vi "Channel Command Engine.vi"(8 "error in":errorcluster, 11 "State Variables":T1={"TCP Refs"={"Connection List"=refnum, "listener ID"=refnum}, "Stop"=refnum, "Top VI"=refnum, "Parameters"={"Properties"={"Name"="", "CAN"={"Database File"=path "", "CAN Interface"=enum."CAN0", "Baud Rate"=0, "Diagnostic Protocol"=enum."GMLAN", "Transport Protocol"=enum."ISO TP - Normal Mode", "Transmit ID"=0, "Receive ID"=0, "Transmit Extension"=0, "Receive Extension"=0, "Receive UUDT ID"=0, "Enable Stream"=TRUE, "VW TP Channel ID"=0, "Security"={"Source DLL Path"=path "", "Security Level"=1, "Target DLL Path"=path ""}, "Fill Frame"=FALSE, "Fill Byte"=255, "Termination"=FALSE}, "FPGA Settings"={"RT Bitfile Path"=path "", "RIO Device"=0, "Enable"=FALSE}, "Reads"=[], "Frames Lookup"=variant, "Writes"=[], "DPIDs"=[], "DPID Lookup"=variant, "DTC descriptor"={"DTC Byte Length"=2, "Status Byte Length"=1, "Add Data Byte Length"=1, "Byte Order"=enum."Motorola"}}, "ChanRefs"={"ToVS.Reads"={"Name"="", "Write to VS Engine FIFO"=refnum, "Pairs"={"Refs"=[], "Values"=[]}}, "ToVS.DTCs"={"Name"="", "Write to VS Engine FIFO"=refnum, "Pairs"={"Refs"=[], "Values"=[]}}, "ToVS.DTCCount"={"Name"="", "Write to VS Engine FIFO"=refnum, "Pairs"={"Refs"=[], "Values"=[]}}, "ToVS.Status"={"Name"="", "Write to VS Engine FIFO"=refnum, "Pairs"={"Refs"=[], "Values"=[]}}, "FromVS.Writes"={"Name"="", "Read from VS Engine FIFO"=refnum, "Pairs"={"Refs"=[], "Values"=[]}}, "Cmds"={"Name"="", "Write to VS Engine FIFO"=refnum, "Read from VS Engine FIFO"=refnum, "Pairs"={"Chan Refs"=[], "Prev. Values"=[]}}}}, "ADCS Connection"={"Diag CAN Handle"=0, "Transport Protocol"=enum."ISO TP - Normal Mode", "Receive Address Extension"=0, "Transmit Address Extension"=0, "Receive CAN Id"=0, "Transmit CAN Id"=0, "Diag CAN Queue"=refnum, "Log Frames ?"=FALSE, "My TP Address"=0, "Other TP Address"=0, "T1"=0, "T2"=0, "T3"=0, "T4"=0, "Tx SN"=0, "Block Size"=0, "Rx SN"=0, "VW TP Initialized?"=FALSE, "Tx block no"=0, "baud rate"=0, "Interface"="", "Channel Diag CAN Handle"=0, "UDP Connection ID"=refnum, "TCP Connection ID"=refnum, "Target IP Addr"=0, "Source Address"=0, "Target Address"=0, "Send Header NACK?"=FALSE, "DLL Handle"=0, "NAD"=0, "Time Stamp read first"=0.0, "Time Stamp read last"=0.0, "Time Stamp write first"=0.0, "Time Stamp write last"=0.0, "Time Stamp write"=0.0, "Time Stamp read"=0.0}, "XNET References"={"Database"="", "GMLAN DPID Session"="", "Cluster"=""}, "BufferedCmds"=refnum, "XNETEngine (GMLAN)"=refnum} {"Parameters"."ChanRefs"."Cmds"."Pairs"."Chan Refs" format="%.0x"; "Parameters"."ChanRefs"."ToVS.Status"."Pairs"."Refs" format="%.0x"; "Parameters"."ChanRefs"."ToVS.DTCCount"."Pairs"."Refs" format="%.0x"; "Parameters"."ChanRefs"."ToVS.DTCs"."Pairs"."Refs" format="%.0x"; "Parameters"."ChanRefs"."ToVS.Reads"."Pairs"."Refs" format="%.0x"; "Parameters"."Properties"."Writes"."Signals"."Byte Order" items=["Little Endian", "Big Endian"]; "Parameters"."Properties"."Writes"."Signals"."Data Type" items=["Signed", "Unsigned", "IEEE Float"]; "Parameters"."Properties"."CAN"."Fill Byte" format="%.0x"; "Parameters"."Properties"."CAN"."VW TP Channel ID" format="%.0x"; "Parameters"."Properties"."CAN"."Receive UUDT ID" format="%.0x"; "Parameters"."Properties"."CAN"."Receive Extension" format="%.0x"; "Parameters"."Properties"."CAN"."Transmit Extension" format="%.0x"; "Parameters"."Properties"."CAN"."Receive ID" format="%.0x"; "Parameters"."Properties"."CAN"."Transmit ID" format="%.0x"; "Parameters"."Properties"."Reads"."Signals"."Byte Order" items=["Little Endian", "Big Endian"]; "Parameters"."Properties"."Reads"."Signals"."Data Type" items=["Signed", "Unsigned", "IEEE Float"]}) -> (0 "error out":errorcluster)   [LabVIEW 2015, in "Diagnostics Addon Engine.lvlib"]
uses:
  Diagnostics Addon Engine.lvlib
  Types/State Variables.ctl
  Types/TCP Refs.ctl
  STM/STM Lookup Table Ref.ctl
  Stop FG/Stop Global Ref.ctl
  Types/Main Configuration.ctl
  Shared/Types/Section Properties.ctl
  Shared/Types/CAN Configuration.ctl
  Shared/Types/CAN Interface.ctl
  Shared/Types/Diagnostic Protocols.ctl
  Shared/Types/Transport Protocols.ctl
  Shared/Types/Security.ctl
  Shared/Types/FPGA Bitfile Settings.ctl
  Shared/Types/Common Frame Parameters.ctl
  Shared/Types/MessageType Selector.ctl
  Shared/Types/Signal Parameters.ctl
  Shared/Types/DPID Parameters.ctl
  Shared/Types/DPID Periodic Rate.ctl
  Shared/Types/DTC Descriptor Parameters.ctl
  Types/VS Data Channels.ctl
  Inline Async API/Controls/Write To VS Engine.ctl
  <vilib>/NI Veristand/Custom Device API/Data Reference.ctl
  Inline Async API/Controls/Read From VS Engine.ctl
  <vilib>/NI Veristand/Custom Device API/Block Data Reference.ctl
  Inline Async API/Controls/ReadWrite Data.ctl
  <vilib>/Automotive Diagnostic Command Set/Diagnostic Transport.llb/Diag Reference.ctl
  <vilib>/Automotive Diagnostic Command Set/Diagnostic Transport.llb/Transport Protocol Selector.ctl
  <vilib>/Automotive Diagnostic Command Set/Diagnostic Transport.llb/Diag CAN Frame Log.ctl
  Types/XNET References.ctl
  <vilib>/NI/AMC/Message Queue.ctl
  <vilib>/NI/AMC/Message.ctl
  <vilib>/NI/Tools/Keyed Array/KeyedArray.ctl
  Stop FG/Stop Global Commands.ctl
  Shared/Types/Channel Commands Enum.ctl
  Shared/Types/Memory Command Parameters.ctl
  Shared/Types/PassThru Channel Based Command Parameters.ctl
  Shared/Types/ReadDTCbyDTCNumber Parameters.ctl
  Shared/Types/Communication Parameters.ctl
  Shared/Types/Input Output Cmd Parameters.ctl
  GMLAN/_SubVIs/ReadFailureRecordData_readFailureRecordParameters_failureRecordIdentifier.ctl
  <vilib>/NI/AMC/Update Message Routing Info.vi
  <vilib>/NI/AMC/Create Multiple Messages.vi
  <vilib>/NI/AMC/Create Single Message.vi
  <vilib>/NI/AMC/Send Message.vi
  Error Handling API/Error Handling API.lvlib
  Stop FG/Stop FG.lvlib
  Shared/Diagnostics Addon Shared.lvlib
  <vilib>/NI/AMC/AMC.lvlib
  GMLAN/GMLAN.lvlib
  <vilib>/NI Veristand/Custom Device API/Custom Device API.lvlib
  <vilib>/NI/Tools/Keyed Array/Tools_KeyedArray.lvlib
  <vilib>/addons/Automotive Diagnostic Command Set/NI_Automotive Diagnostic Command Set.lvlib
  Inline Async API/Inline Async API.lvlib
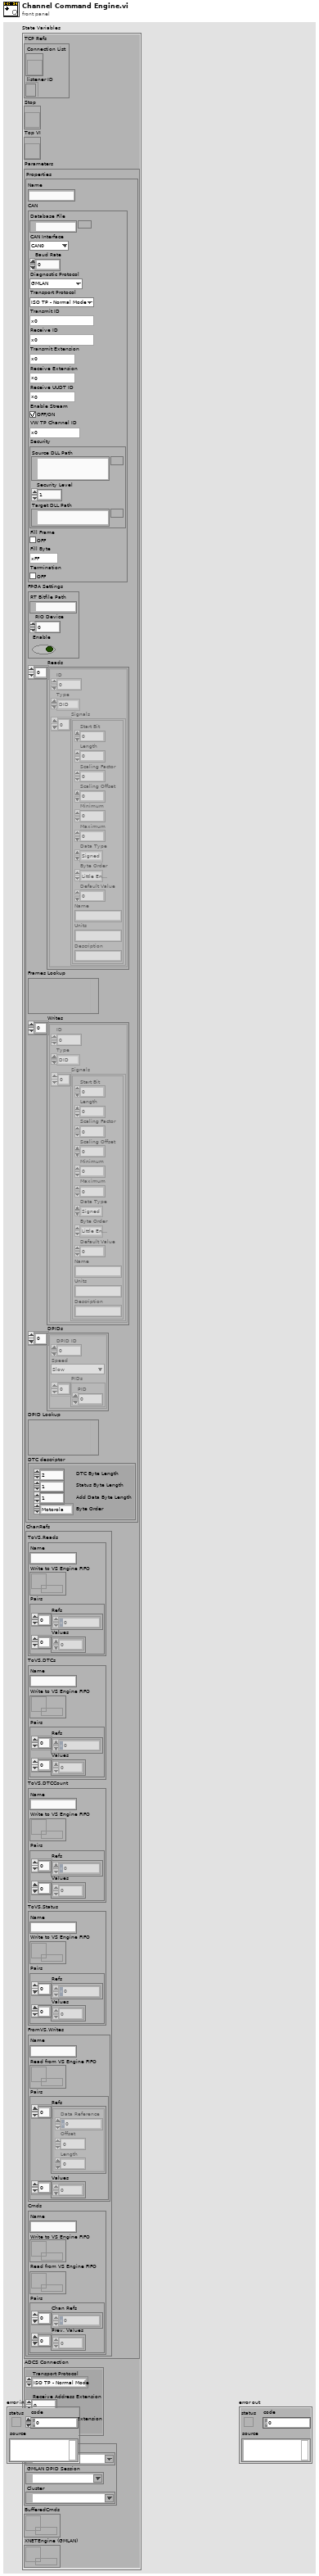
[diagram p1: front panel]
types:
  T1 = typedef "Diagnostics Addon Engine.lvlib/State Variables.ctl" = cluster{"TCP Refs":T2, "Stop":T4, "Top VI":refnum<vi>, "Parameters":T5, "ADCS Connection":T25, "XNET References":T27, "BufferedCmds":T28, "XNETEngine (GMLAN)":T28}
  T2 = typedef "Diagnostics Addon Engine.lvlib/TCP Refs.ctl" = cluster{"Connection List":T3, "listener ID":refnum<k5>}
  T3 = typedef "Diagnostics Addon Engine.lvlib/STM Lookup Table Ref.ctl" = refnum<vi>
  T4 = typedef "Diagnostics Addon Engine.lvlib/Stop FG.lvlib/Stop Global Ref.ctl" = refnum<vi>
  T5 = typedef "Diagnostics Addon Engine.lvlib/Main Configuration.ctl" = cluster{"Properties":T6, "ChanRefs":T19}
  T6 = typedef "Diagnostics Addon Shared.lvlib/Section Properties.ctl" = cluster{"Name":string, "CAN":T7, "FPGA Settings":T12, "Reads":T13[], "Frames Lookup":variant, "Writes":T13[], "DPIDs":T16[], "DPID Lookup":variant, "DTC descriptor":T18}
  T7 = typedef "Diagnostics Addon Shared.lvlib/CAN Configuration.ctl" = cluster{"Database File":path, "CAN Interface":T8, "Baud Rate":u32, "Diagnostic Protocol":T9, "Transport Protocol":T10, "Transmit ID":u32, "Receive ID":u32, "Transmit Extension":u8, "Receive Extension":u8, "Receive UUDT ID":u32, "Enable Stream":bool, "VW TP Channel ID":u32, "Security":T11, "Fill Frame":bool, "Fill Byte":u8, "Termination":bool}
  T8 = typedef "Diagnostics Addon Shared.lvlib/CAN Interface.ctl" = enum16{"CAN0", "CAN1", "CAN2", "CAN3", "CAN4", "CAN5", "CAN6", "CAN7", "CAN8", "CAN9", "CAN10", "CAN11", "CAN12", "CAN13", "CAN14", "CAN15", "CAN16", "CAN17", "CAN18", "CAN19", "CAN20", "CAN21", "CAN22", "CAN23", "CAN24", "CAN25", "CAN26", "CAN27", "CAN28", "CAN29", "CAN30", "CAN31", "CAN32", "CAN33", "CAN34", "CAN35", "CAN36", "CAN37", "CAN38", "CAN39", "CAN40", "CAN41", "CAN42", "CAN43", "CAN44", "CAN45", "CAN46", "CAN47", "CAN48", "CAN49", "CAN50", "CAN51", "CAN52", "CAN53", "CAN54", "CAN55", "CAN56", "CAN57", "CAN58", "CAN59", "CAN60", "CAN61", "CAN62", "CAN63", "CAN 256 (Virtual)", "CAN 257 (Virtual)"}
  T9 = typedef "Diagnostics Addon Shared.lvlib/Diagnostic Protocols.ctl" = enum16{"GMLAN", "KWP-2000", "UDS"}
  T10 = typedef "Diagnostics Addon Shared.lvlib/Transport Protocols.ctl" = enum16{"ISO TP - Normal Mode", "ISO TP - Mixed Mode", "VW TP 2.0", "Diagnostics on IP"}
  T11 = typedef "Diagnostics Addon Shared.lvlib/Security.ctl" = cluster{"Source DLL Path":path, "Security Level":u8, "Target DLL Path":path}
  T12 = typedef "Diagnostics Addon Shared.lvlib/FPGA Bitfile Settings.ctl" = cluster{"RT Bitfile Path":path, "RIO Device":u16, "Enable":bool}
  T13 = typedef "Diagnostics Addon Shared.lvlib/Common Frame Parameters.ctl" = cluster{"ID":u32, "Type":T14, "Signals":T15[]}
  T14 = typedef "Diagnostics Addon Shared.lvlib/MessageType Selector.ctl" = enum16{"DID", "CDID", "PID", "CPID", "Write Memory", "Read Memory", "DTC Control", "IO Cmd", "IO Resp", "Routine Start Cmd", "Routine Start Resp", "Routine Status Cmd", "Routine Status Resp", "Routine Stop Cmd", "Routine Stop Resp"}
  T15 = typedef "Diagnostics Addon Shared.lvlib/Signal Parameters.ctl" = cluster{"Start Bit":u8, "Length":u8, "Scaling Factor":dbl, "Scaling Offset":dbl, "Minimum":dbl, "Maximum":dbl, "Data Type":u32, "Byte Order":u32, "Default Value":dbl, "Name":string, "Units":string, "Description":string}
  T16 = typedef "Diagnostics Addon Shared.lvlib/DPID Parameters.ctl" = cluster{"DPID ID":u8, "Speed":T17, "PIDs":u16[]}
  T17 = typedef "Diagnostics Addon Shared.lvlib/DPID Periodic Rate.ctl" = enum16{"Slow", "Medium", "Fast"}
  T18 = typedef "Diagnostics Addon Shared.lvlib/DTC Descriptor Parameters.ctl" = cluster{"DTC Byte Length":i32, "Status Byte Length":i32, "Add Data Byte Length":i32, "Byte Order":enum16{"Motorola", "Intel"}}
  T19 = typedef "Diagnostics Addon Engine.lvlib/VS Data Channels.ctl" = cluster{"ToVS.Reads":T20, "ToVS.DTCs":T20, "ToVS.DTCCount":T20, "ToVS.Status":T20, "FromVS.Writes":T22, "Cmds":T24}
  T20 = typedef "Diagnostics Addon Engine.lvlib/Inline Async API.lvlib/Write To VS Engine.ctl" = cluster{"Name":string, "Write to VS Engine FIFO":refnum<k33>, "Pairs":cluster{"Refs":T21[], "Values":dbl[]}}
  T21 = typedef "Custom Device API.lvlib/Data Reference.ctl" = i32
  T22 = typedef "Diagnostics Addon Engine.lvlib/Inline Async API.lvlib/Read From VS Engine.ctl" = cluster{"Name":string, "Read from VS Engine FIFO":refnum<k33>, "Pairs":cluster{"Refs":T23[], "Values":dbl[]}}
  T23 = typedef "Custom Device API.lvlib/Block Data Reference.ctl" = cluster{"Data Reference":T21, "Offset":u64, "Length":u64}
  T24 = typedef "Diagnostics Addon Engine.lvlib/Inline Async API.lvlib/ReadWrite Data.ctl" = cluster{"Name":string, "Write to VS Engine FIFO":refnum<k33>, "Read from VS Engine FIFO":refnum<k33>, "Pairs":cluster{"Chan Refs":T21[], "Prev. Values":dbl[]}}
  T25 = typedef "NI_Automotive Diagnostic Command Set.lvlib/Diag Reference.ctl" = cluster{"Diag CAN Handle":u32, "Transport Protocol":T26, "Receive Address Extension":u8, "Transmit Address Extension":u8, "Receive CAN Id":u32, "Transmit CAN Id":u32, "Diag CAN Queue":refnum<queue>, "Log Frames ?":bool, "My TP Address":u8, "Other TP Address":u8, "T1":u16, "T2":u16, "T3":u16, "T4":u16, "Tx SN":u8, "Block Size":u8, "Rx SN":u8, "VW TP Initialized?":bool, "Tx block no":u8, "baud rate":u32, "Interface":string, "Channel Diag CAN Handle":u32, "UDP Connection ID":refnum<k16>, "TCP Connection ID":refnum<k5>, "Target IP Addr":u32, "Source Address":u16, "Target Address":u16, "Send Header NACK?":bool, "DLL Handle":u32, "NAD":u8, "Time Stamp read first":dbl, "Time Stamp read last":dbl, "Time Stamp write first":dbl, "Time Stamp write last":dbl, "Time Stamp write":dbl, "Time Stamp read":dbl}
  T26 = typedef "NI_Automotive Diagnostic Command Set.lvlib/Transport Protocol Selector.ctl" = enum16{"ISO TP - Normal Mode", "ISO TP - Mixed Mode", "VW TP 2.0", "Diagnostics on IP", "ISO TP LIN"}
  T27 = typedef "Diagnostics Addon Engine.lvlib/XNET References.ctl" = cluster{"Database":refnum<k21>, "GMLAN DPID Session":refnum<k21>, "Cluster":refnum<k21>}
  T28 = typedef "AMC.lvlib/Message Queue.ctl" = refnum<queue>
  T29 = typedef "Diagnostics Addon Engine.lvlib/Stop FG.lvlib/Stop Global Commands.ctl" = enum16{"Write", "Read", "Reset"}
  T30 = typedef "Diagnostics Addon Shared.lvlib/Channel Commands Enum.ctl" = enum8{"None", "EnableDiagnosticSession", "DisableDiagnosticSession", "ReadDataIdentifiers", "ReadDataIdentifier", "WriteDataIndentifier", "ReadPIDsOnDemand", "ReadPIDOnDemand", "WriteCPID", "WriteMemory", "ReadMemory", "ReadDTCs", "ClearDTCs", "ControlDTC", "ForceTesterPresent", "DisableNormalCommunication", "ReturnToNormalMode", "InputOutputControl", "StartRoutine", "RequestRoutineStatus", "StopRoutine", "ECUReset", "UnlockECU", "ClearSuccessBit", "ConfigureandStartPIDs", "StopPIDs", "StartDTCs", "EnableChangeDTCCount", "DisableChangeDTCCount", "ReadFailureRecordParameters", "PassThru Channel Based"}
  T31 = typedef "Diagnostics Addon Shared.lvlib/Memory Command Parameters.ctl" = cluster{"Address":u64, "Service Type":u32, "Address Length":u8, "Size Length":u8}
  T32 = typedef "Diagnostics Addon Shared.lvlib/PassThru Channel Based Command Parameters.ctl" = cluster{"Service":u64, "Service Length":u8, "Data Length":u32, "Response Required":bool}
  T33 = typedef "Diagnostics Addon Shared.lvlib/ReadDTCbyDTCNumber Parameters.ctl" = cluster{"DTC":u16, "FailTypeByte":u8}
  T34 = typedef "Diagnostics Addon Shared.lvlib/Communication Parameters.ctl" = cluster{"Type":u8, "CommType":u8}
  T35 = typedef "Diagnostics Addon Shared.lvlib/Input Output Cmd Parameters.ctl" = cluster{"ID":u16, "Mode":u8}
  T36 = typedef "GMLAN.lvlib/ReadFailureRecordData_readFailureRecordParameters_failureRecordIdentifier.ctl" = cluster{"failureRecordNumber":u8, "DTC ID":u16, "DTCFailureType":u8}
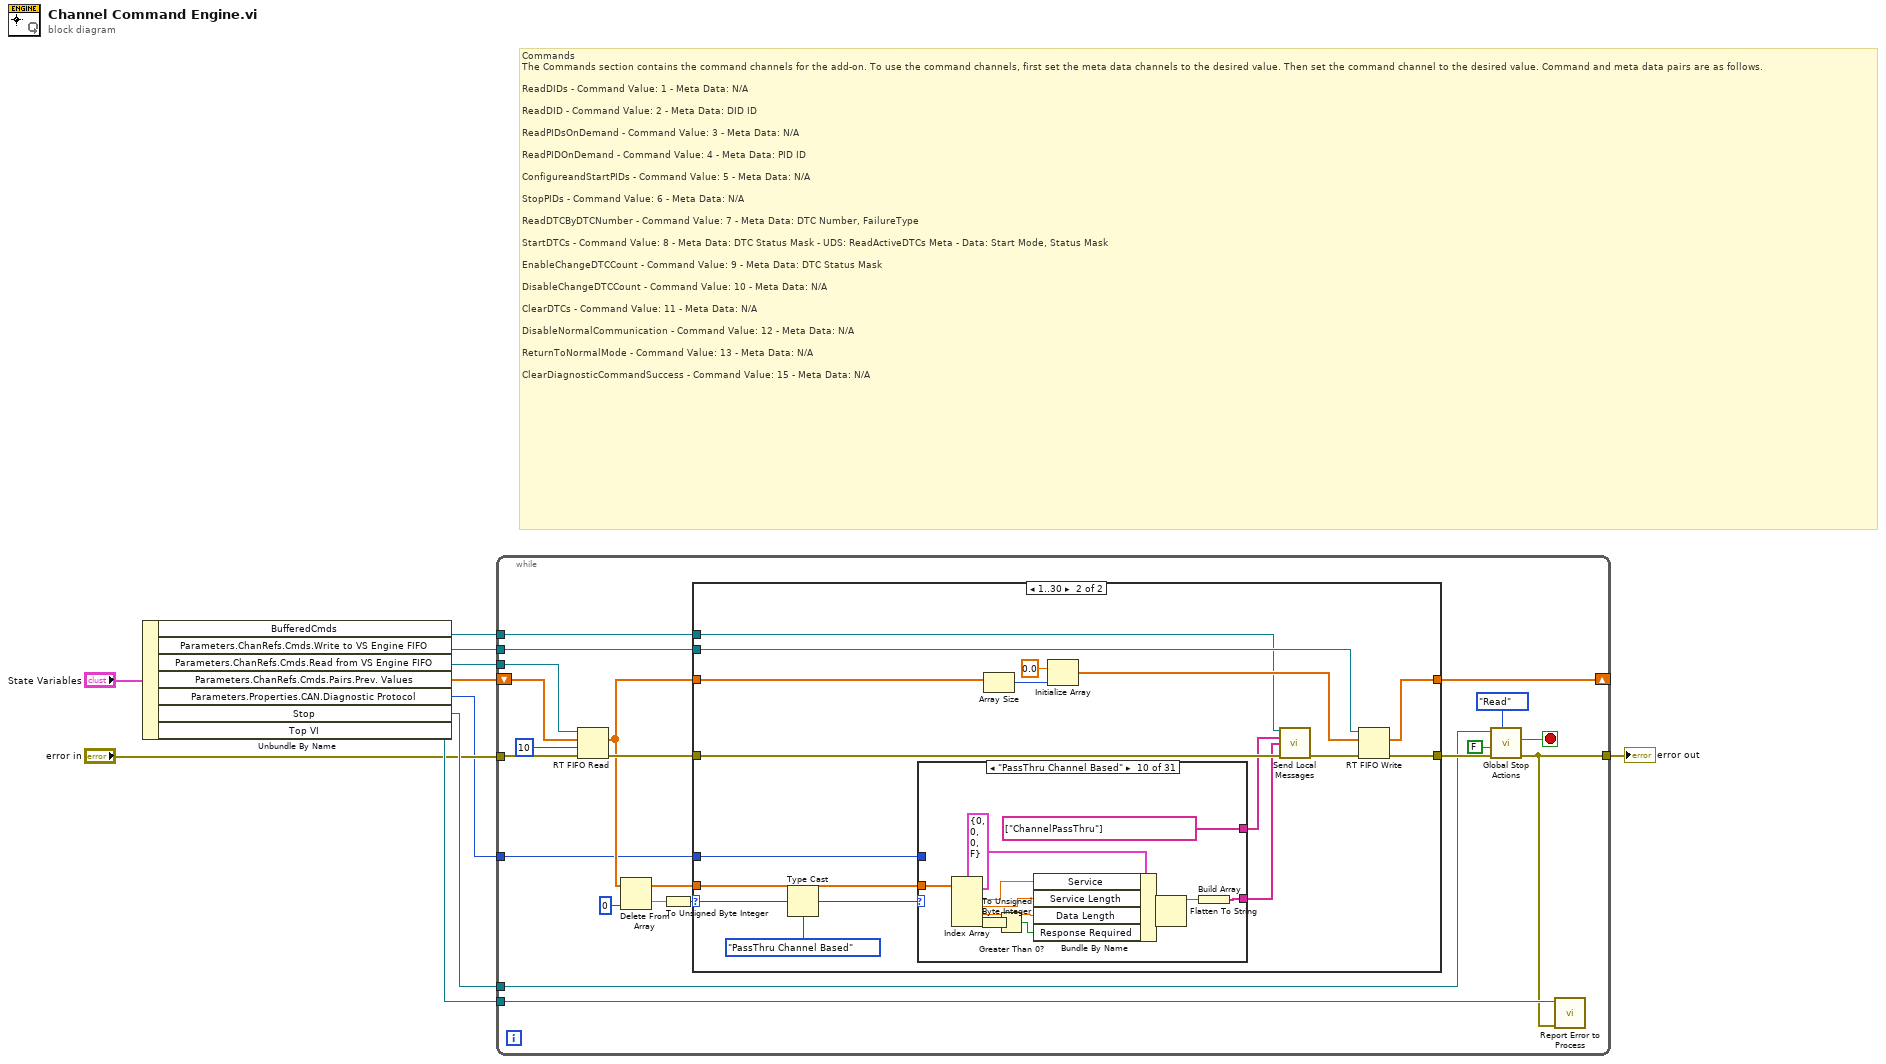
[diagram p0: block diagram]
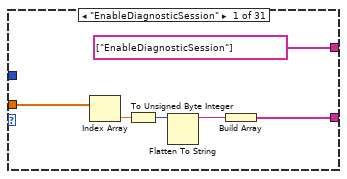
[diagram p3: hidden frame]
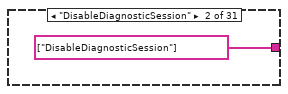
[diagram p4: hidden frame]
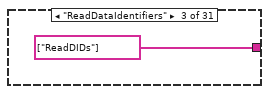
[diagram p5: hidden frame]
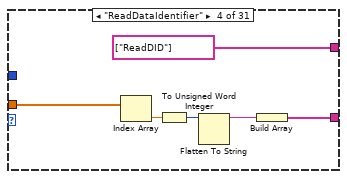
[diagram p6: hidden frame]
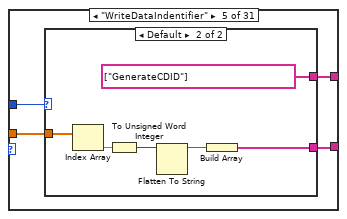
[diagram p7: hidden frame]
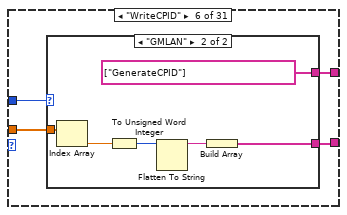
[diagram p9: hidden frame]
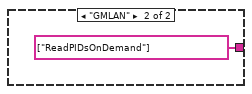
[diagram p12: hidden frame]
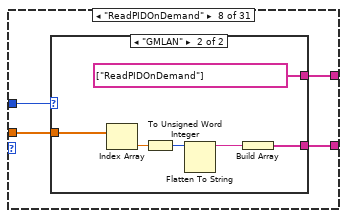
[diagram p13: hidden frame]
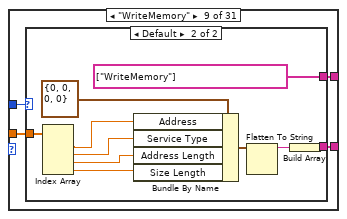
[diagram p15: hidden frame]
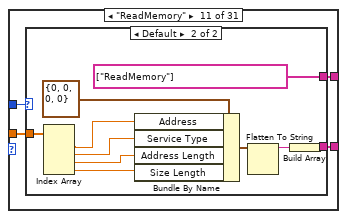
[diagram p17: hidden frame]
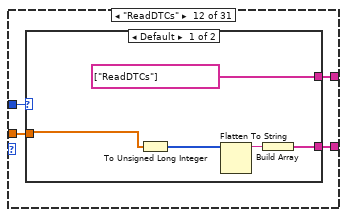
[diagram p19: hidden frame]
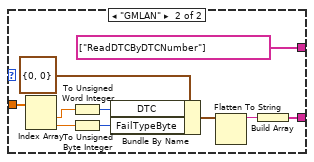
[diagram p20: hidden frame]
diagram:
  # "Commands\nThe Commands section contains the command channels for the add-on. To use the command channels, first set the meta data channels to the desired value. Then set the command channel to the desired value. Command and meta data pairs are as follows.\n\nReadDIDs - Command Value: 1 - Meta Data: N/A\n\nReadDID - Command Value: 2 - Meta Data: DID ID\n\nReadPIDsOnDemand - Command Value: 3 - Meta Data: N/A\n\nReadPIDOnDemand - Command Value: 4 - Meta Data: PID ID\n\nConfigureandStartPIDs - Command Value: 5 - Meta Data: N/A\n\nStopPIDs - Command Value: 6 - Meta Data: N/A\n\nReadDTCByDTCNumber - Command Value: 7 - Meta Data: DTC Number, FailureType\n\nStartDTCs - Command Value: 8 - Meta Data: DTC Status Mask - UDS: ReadActiveDTCs Meta - Data: Start Mode, Status Mask\n\nEnableChangeDTCCount - Command Value: 9 - Meta Data: DTC Status Mask\n\nDisableChangeDTCCount - Command Value: 10 - Meta Data: N/A\n\nClearDTCs - Command Value: 11 - Meta Data: N/A\n\nDisableNormalCommunication - Command Value: 12 - Meta Data: N/A\n\nReturnToNormalMode - Command Value: 13 - Meta Data: N/A\n\nClearDiagnosticCommandSuccess - Command Value: 15 - Meta Data: N/A"
  n1 = Unbundle By Name("State Variables") -> ("BufferedCmds"=w2:T28, "Parameters.ChanRefs.Cmds.Write to VS Engine FIFO"=w3:refnum<k33>, "Parameters.ChanRefs.Cmds.Read from VS Engine FIFO"=w5:refnum<k33>, "Parameters.ChanRefs.Cmds.Pairs.Prev. Values"=w4:dbl[], "Parameters.Properties.CAN.Diagnostic Protocol"=w1:T9, "Stop"=w9:T4, "Top VI"=w8:refnum<vi>)
  n2 = while {
    tunnel: w5 -> [w25]
    shift-right: [w23] -> _
    shift-left: w4 -> [w24]
    tunnel: w9 -> [w18]
    tunnel: w8 -> [w17]
    tunnel: [w16] -> w7
    tunnel: "error in" -> [w14]
    tunnel: w3 -> [w13]
    tunnel: w2 -> [w12]
    tunnel: w1 -> [w11]
    stop <- w15 stop-if-true
    n3 = RT FIFO Read(0:w25, 1:w24, 2:10 ("timeout in ms (0)"), 3:w14) -> (9:w26:dbl[], 11:w31:errorcluster)  [unwired: 3 out]
    n4 = Delete From Array(array=w26, index=0) -> (deleted portion=w29:dbl, array with subset deleted=w27:dbl[])  [unwired: 1 in]
    n5 = To Unsigned Byte Integer(number=w29) -> (unsigned 8bit integer=w28:u8)
    n6 = case shown="1..30" w28 {
      selector: w28 -> [_ w34]
      tunnel: w31 -> [w32 w45]
      tunnel: w27 -> [_ w43]
      tunnel: w26 -> [w33 w49]
      tunnel: [w33 w39] -> w23
      tunnel: [w32 w46] -> w19
      tunnel: w13 -> [_ w40]
      tunnel: w12 -> [_ w36]
      tunnel: w11 -> [_ w35]
      frame 0, Default {
      }
      frame 1..30 {
        n7 = Type Cast(type=Channel_Commands_Enum."PassThru Channel Based", x=w34) -> (*(type *) &x=w38:T30)
        n8 = case shown="\"PassThru Channel Based\"" w38 {
          tunnel: w43 -> [w51 _ _ w59 w66 w76 _ w89 w98 w121 w124 w139 w157 w163 w173 w176 _ w187 w201 w211 w221 w232 _ _ _ _ w250 w260 _ w276 _]
          tunnel: [string[] ["EnableDiagnosticSession"] string[] ["DisableDiagnosticSession"] string[] ["ReadDIDs"] string[] ["ReadDID"] w67 w77 w85 w90 w100 string[] ["ChannelPassThru"] w126 w140 string[] ["ClearDTCs"] string[] ["ControlDTC"] string[] ["ForceTesterPresent"] string[] ["DisableNormalCommunication"] string[] ["ReturnToNormalMode"] w189 w203 w213 w223 w233 string[] ["UnlockECU"] string[] ["ClearSuccessBit"] w243 w246 w251 w261 w270 w278 _] -> w42
          tunnel: [w50 _ _ w58 w65 w75 _ w88 w97 w120 w123 w138 w156 w162 w172 w175 _ w186 w200 w210 w220 w231 _ _ _ _ w249 w259 w269 w277 _] -> w41
          tunnel: w35 -> [_ _ _ _ w64 w74 w84 w87 w99 _ w125 w137 _ _ _ _ _ w188 w202 w212 w222 w230 _ _ w242 w245 w248 w258 w268 w275 _]
          frame "EnableDiagnosticSession" {
            n9 = Index Array(array=w51) -> (element=w54:dbl)  [unwired: 1 in]
            n10 = To Unsigned Byte Integer(number=w54) -> (unsigned 8bit integer=w53:u8)
            n11 = Flatten To String(anything=w53) -> (data string=w52:string)  [unwired: 3 in, 2 out]
            n12 = Build Array(w52) -> (w50:string[])
          }
          frame "DisableDiagnosticSession" {
          }
          frame "ReadDataIdentifiers" {
          }
          frame "ReadDataIdentifier" {
            n13 = Index Array(array=w59) -> (element=w62:dbl)  [unwired: 1 in]
            n14 = To Unsigned Word Integer(number=w62) -> (unsigned 16bit integer=w61:u16)
            n15 = Flatten To String(anything=w61) -> (data string=w60:string)  [unwired: 3 in, 2 out]
            n16 = Build Array(w60) -> (w58:string[])
          }
          frame "WriteDataIndentifier" {
            n17 = case shown="Default" w64 {
              tunnel: [_ string[] ["GenerateCDID"]] -> w67
              tunnel: w66 -> [_ w72]
              tunnel: [_ w71] -> w65
              frame "GMLAN" {
              }
              frame Default {
                n18 = Index Array(array=w72) -> (element=w70:dbl)  [unwired: 1 in]
                n19 = To Unsigned Word Integer(number=w70) -> (unsigned 16bit integer=w68:u16)
                n20 = Flatten To String(anything=w68) -> (data string=w69:string)  [unwired: 3 in, 2 out]
                n21 = Build Array(w69) -> (w71:string[])
              }
            }
          }
          frame "WriteCPID" {
            n22 = case shown="\"GMLAN\"" w74 {
              tunnel: [_ string[] ["GenerateCPID"]] -> w77
              tunnel: w76 -> [_ w82]
              tunnel: [_ w81] -> w75
              frame Default {
              }
              frame "GMLAN" {
                n23 = Index Array(array=w82) -> (element=w80:dbl)  [unwired: 1 in]
                n24 = To Unsigned Word Integer(number=w80) -> (unsigned 16bit integer=w78:u16)
                n25 = Flatten To String(anything=w78) -> (data string=w79:string)  [unwired: 3 in, 2 out]
                n26 = Build Array(w79) -> (w81:string[])
              }
            }
          }
          frame "ReadPIDsOnDemand" {
            n27 = case shown="Default" w84 {
              tunnel: [_ string[] ["ReadPIDsOnDemand"]] -> w85
              frame Default {
              }
              frame "GMLAN" {
              }
            }
          }
          frame "ReadPIDOnDemand" {
            n28 = case shown="\"GMLAN\"" w87 {
              tunnel: [_ string[] ["ReadPIDOnDemand"]] -> w90
              tunnel: w89 -> [_ w92]
              tunnel: [_ w91] -> w88
              frame Default {
              }
              frame "GMLAN" {
                n29 = Index Array(array=w92) -> (element=w95:dbl)  [unwired: 1 in]
                n30 = To Unsigned Word Integer(number=w95) -> (unsigned 16bit integer=w94:u16)
                n31 = Flatten To String(anything=w94) -> (data string=w93:string)  [unwired: 3 in, 2 out]
                n32 = Build Array(w93) -> (w91:string[])
              }
            }
          }
          frame "WriteMemory" {
            n33 = case shown="Default" w99 {
              tunnel: [_ string[] ["WriteMemory"]] -> w100
              tunnel: w98 -> [_ w102]
              tunnel: [_ w109] -> w97
              frame "GMLAN" {
              }
              frame Default {
                n34 = Index Array(array=w102) -> (element #1=w106:dbl, element #2=w107:dbl, element #3=w105:dbl, element #4=w104:dbl)  [unwired: 4 in]
                n35 = Bundle By Name(cluster=T31 {"Address"=0, "Service Type"=0, "Address Length"=0, "Size Length"=0}, "Address"=w106, "Service Type"=w107, "Address Length"=w105, "Size Length"=w104) -> (w108:T31)
                n36 = Flatten To String(anything=w108) -> (data string=w103:string)  [unwired: 3 in, 2 out]
                n37 = Build Array(w103) -> (w109:string[])
              }
            }
          }
          frame "PassThru Channel Based" {
            n38 = Index Array(array=w121) -> (element #1=w117:dbl, element #2=w118:dbl, element #3=w116:dbl, element #4=w113:dbl)  [unwired: 4 in]
            n39 = To Unsigned Byte Integer(number=w113) -> (unsigned 8bit integer=w112:u8)
            n40 = Greater Than 0?(x=w112) -> (x > 0?=w111:bool)
            n41 = Bundle By Name(cluster=T32 {"Service"=0, "Service Length"=0, "Data Length"=0, "Response Required"=FALSE}, "Service"=w117, "Service Length"=w118, "Data Length"=w116, "Response Required"=w111) -> (w119:T32)
            n42 = Flatten To String(anything=w119) -> (data string=w115:string)  [unwired: 3 in, 2 out]
            n43 = Build Array(w115) -> (w120:string[])
          }
          frame "ReadMemory" {
            n44 = case shown="Default" w125 {
              tunnel: [_ string[] ["ReadMemory"]] -> w126
              tunnel: w124 -> [_ w135]
              tunnel: [_ w133] -> w123
              frame "GMLAN" {
              }
              frame Default {
                n45 = Index Array(array=w135) -> (element #1=w129:dbl, element #2=w130:dbl, element #3=w128:dbl, element #4=w127:dbl)  [unwired: 4 in]
                n46 = Bundle By Name(cluster=T31 {"Address"=0, "Service Type"=0, "Address Length"=0, "Size Length"=0}, "Address"=w129, "Service Type"=w130, "Address Length"=w128, "Size Length"=w127) -> (w131:T31)
                n47 = Flatten To String(anything=w131) -> (data string=w134:string)  [unwired: 3 in, 2 out]
                n48 = Build Array(w134) -> (w133:string[])
              }
            }
          }
          frame "ReadDTCs" {
            n49 = case shown="Default" w137 {
              tunnel: [string[] ["ReadDTCs"] string[] ["ReadDTCByDTCNumber"]] -> w140
              tunnel: w139 -> [w143 w152]
              tunnel: [w141 w151] -> w138
              frame Default {
                n50 = To Unsigned Long Integer(number=w143) -> (unsigned 32bit integer=w145:u32[])
                n51 = Flatten To String(anything=w145) -> (data string=w144:string)  [unwired: 3 in, 2 out]
                n52 = Build Array(w144) -> (w141:string[])
              }
              frame "GMLAN" {
                n53 = Index Array(array=w152) -> (element #1=w154:dbl, element #2=w150:dbl)  [unwired: 2 in]
                n54 = To Unsigned Word Integer(number=w154) -> (unsigned 16bit integer=w147:u16)
                n55 = To Unsigned Byte Integer(number=w150) -> (unsigned 8bit integer=w149:u8)
                n56 = Bundle By Name(cluster=T33 {"DTC"=0, "FailTypeByte"=0}, "DTC"=w147, "FailTypeByte"=w149) -> (w146:T33)
                n57 = Flatten To String(anything=w146) -> (data string=w153:string)  [unwired: 3 in, 2 out]
                n58 = Build Array(w153) -> (w151:string[])
              }
            }
          }
          frame "ClearDTCs" {
            n59 = Index Array(array=w157) -> (element=w160:dbl)  [unwired: 1 in]
            n60 = To Unsigned Long Integer(number=w160) -> (unsigned 32bit integer=w159:u32)
            n61 = Flatten To String(anything=w159) -> (data string=w158:string)  [unwired: 3 in, 2 out]
            n62 = Build Array(w158) -> (w156:string[])
          }
          frame "ControlDTC" {
            n63 = Index Array(array=w163) -> (element=w166:dbl)  [unwired: 1 in]
            n64 = To Unsigned Long Integer(number=w166) -> (unsigned 32bit integer=w165:u32)
            n65 = Flatten To String(anything=w165) -> (data string=w164:string)  [unwired: 3 in, 2 out]
            n66 = Build Array(w164) -> (w162:string[])
          }
          frame "ForceTesterPresent" {
            n67 = Index Array(array=w173) -> (element=w171:dbl)  [unwired: 1 in]
            n68 = To Unsigned Byte Integer(number=w171) -> (unsigned 8bit integer=w168:u8)
            n69 = Number To Boolean Array(number=w168) -> (Boolean array=w169:bool[])
            n70 = Flatten To String(anything=w169) -> (data string=w170:string)  [unwired: 3 in, 2 out]
            n71 = Build Array(w170) -> (w172:string[])
          }
          frame "DisableNormalCommunication" {
            n72 = Index Array(array=w176) -> (element #1=w181:dbl, element #2=w182:dbl)  [unwired: 2 in]
            n73 = To Unsigned Byte Integer(number=w182) -> (unsigned 8bit integer=w179:u8)
            n74 = To Unsigned Byte Integer(number=w181) -> (unsigned 8bit integer=w180:u8)
            n75 = Bundle By Name(cluster=T34 {"Type"=0, "CommType"=0} ("Cluster"), "Type"=w180, "CommType"=w179) -> (w178:T34)
            n76 = Flatten To String(anything=w178) -> (data string=w183:string)  [unwired: 3 in, 2 out]
            n77 = Build Array(w183) -> (w175:string[])
          }
          frame "ReturnToNormalMode" {
          }
          frame "InputOutputControl" {
            n78 = case shown="Default" w188 {
              tunnel: [_ string[] ["InputOutputControl"]] -> w189
              tunnel: w187 -> [_ w197]
              tunnel: [_ w190] -> w186
              frame "GMLAN" {
              }
              frame Default {
                n79 = Index Array(array=w197) -> (element #1=w195:dbl, element #2=w196:dbl)  [unwired: 2 in]
                n80 = To Unsigned Byte Integer(number=w196) -> (unsigned 8bit integer=w192:u8)
                n81 = To Unsigned Word Integer(number=w195) -> (unsigned 16bit integer=w193:u16)
                n82 = Bundle By Name(cluster=T35 {"ID"=0, "Mode"=0}, "ID"=w193, "Mode"=w192) -> (w191:T35)
                n83 = Flatten To String(anything=w191) -> (data string=w198:string)  [unwired: 3 in, 2 out]
                n84 = Build Array(w198) -> (w190:string[])
              }
            }
          }
          frame "StartRoutine" {
            n85 = case shown="Default" w202 {
              tunnel: [_ string[] ["StartRoutine"]] -> w203
              tunnel: w201 -> [_ w208]
              tunnel: [_ w204] -> w200
              frame "GMLAN" {
              }
              frame Default {
                n86 = Index Array(array=w208) -> (element=w207:dbl)  [unwired: 1 in]
                n87 = To Unsigned Word Integer(number=w207) -> (unsigned 16bit integer=w205:u16)
                n88 = Flatten To String(anything=w205) -> (data string=w206:string)  [unwired: 3 in, 2 out]
                n89 = Build Array(w206) -> (w204:string[])
              }
            }
          }
          frame "RequestRoutineStatus" {
            n90 = case shown="Default" w212 {
              tunnel: [_ string[] ["RequestRoutineStatus"]] -> w213
              tunnel: w211 -> [_ w215]
              tunnel: [_ w214] -> w210
              frame "GMLAN" {
              }
              frame Default {
                n91 = Index Array(array=w215) -> (element=w218:dbl)  [unwired: 1 in]
                n92 = To Unsigned Word Integer(number=w218) -> (unsigned 16bit integer=w216:u16)
                n93 = Flatten To String(anything=w216) -> (data string=w217:string)  [unwired: 3 in, 2 out]
                n94 = Build Array(w217) -> (w214:string[])
              }
            }
          }
          frame "StopRoutine" {
            n95 = case shown="Default" w222 {
              tunnel: [_ string[] ["StopRoutine"]] -> w223
              tunnel: w221 -> [_ w225]
              tunnel: [_ w224] -> w220
              frame "GMLAN" {
              }
              frame Default {
                n96 = Index Array(array=w225) -> (element=w228:dbl)  [unwired: 1 in]
                n97 = To Unsigned Word Integer(number=w228) -> (unsigned 16bit integer=w226:u16)
                n98 = Flatten To String(anything=w226) -> (data string=w227:string)  [unwired: 3 in, 2 out]
                n99 = Build Array(w227) -> (w224:string[])
              }
            }
          }
          frame "ECUReset" {
            n100 = case shown="Default" w230 {
              tunnel: [_ string[] ["ECUReset"]] -> w233
              tunnel: w232 -> [_ w235]
              tunnel: [_ w234] -> w231
              frame "GMLAN" {
              }
              frame Default {
                n101 = Index Array(array=w235) -> (element=w238:dbl)  [unwired: 1 in]
                n102 = To Unsigned Byte Integer(number=w238) -> (unsigned 8bit integer=w237:u8)
                n103 = Flatten To String(anything=w237) -> (data string=w236:string)  [unwired: 3 in, 2 out]
                n104 = Build Array(w236) -> (w234:string[])
              }
            }
          }
          frame "UnlockECU" {
          }
          frame "ClearSuccessBit" {
          }
          frame "ConfigureandStartPIDs" {
            n105 = case shown="\"GMLAN\"" w242 {
              tunnel: [_ string[] ["ConfigurePIDs", "StartPIDs"]] -> w243
              frame Default {
              }
              frame "GMLAN" {
              }
            }
          }
          frame "StopPIDs" {
            n106 = case shown="\"GMLAN\"" w245 {
              tunnel: [_ string[] ["StopPIDs"]] -> w246
              frame Default {
              }
              frame "GMLAN" {
              }
            }
          }
          frame "StartDTCs" {
            n107 = case shown="\"GMLAN\"" w248 {
              tunnel: [string[] ["StartDTCs"] _] -> w251
              tunnel: w250 -> [w256 _]
              tunnel: [w252 _] -> w249
              frame "GMLAN" {
                n108 = Index Array(array=w256) -> (element=w255:dbl)  [unwired: 1 in]
                n109 = To Unsigned Byte Integer(number=w255) -> (unsigned 8bit integer=w254:u8)
                n110 = Flatten To String(anything=w254) -> (data string=w253:string)  [unwired: 3 in, 2 out]
                n111 = Build Array(w253) -> (w252:string[])
              }
              frame Default {
              }
            }
          }
          frame "EnableChangeDTCCount" {
            n112 = case shown="\"GMLAN\"" w258 {
              tunnel: [_ string[] ["EnableChangeDTCCount"]] -> w261
              tunnel: w260 -> [_ w266]
              tunnel: [_ w262] -> w259
              frame Default {
              }
              frame "GMLAN" {
                n113 = Index Array(array=w266) -> (element=w265:dbl)  [unwired: 1 in]
                n114 = To Unsigned Byte Integer(number=w265) -> (unsigned 8bit integer=w264:u8)
                n115 = Flatten To String(anything=w264) -> (data string=w263:string)  [unwired: 3 in, 2 out]
                n116 = Build Array(w263) -> (w262:string[])
              }
            }
          }
          frame "DisableChangeDTCCount" {
            n117 = case shown="\"GMLAN\"" w268 {
              tunnel: [_ string[] ["DisableChangeDTCCount"]] -> w270
              tunnel: [_ w272] -> w269
              frame Default {
              }
              frame "GMLAN" {
                n118 = Flatten To String(anything=u8 0 ("number")) -> (data string=w273:string)  [unwired: 3 in, 2 out]
                n119 = Build Array(w273) -> (w272:string[])
              }
            }
          }
          frame "ReadFailureRecordParameters" {
            n120 = case shown="\"GMLAN\"" w275 {
              tunnel: [_ string[] ["ReadFailureRecordParameters"]] -> w278
              tunnel: [_ w284] -> w277
              tunnel: w276 -> [_ w283]
              frame Default {
              }
              frame "GMLAN" {
                n121 = Index Array(array=w283) -> (element #1=w289:dbl, element #2=w287:dbl, element #3=w279:dbl)  [unwired: 3 in]
                n122 = To Unsigned Word Integer(number=w289) -> (unsigned 16bit integer=w286:u16)
                n123 = To Unsigned Byte Integer(number=w287) -> (unsigned 8bit integer=w281:u8)
                n124 = To Unsigned Byte Integer(number=w279) -> (unsigned 8bit integer=w280:u8)
                n125 = Bundle By Name(cluster=T36 {"failureRecordNumber"=0, "DTC ID"=0, "DTCFailureType"=0} ("failureRecordIdentifier"), "DTC ID"=w286, "DTCFailureType"=w281, "failureRecordNumber"=w280) -> (w285:T36)
                n126 = Flatten To String(anything=w285) -> (data string=w288:string)  [unwired: 3 in, 2 out]
                n127 = Build Array(w288) -> (w284:string[])
              }
            }
          }
          frame "None", Default {
          }
        }
        n128 = Array Size(array=w49) -> (size(s)=w48:i32)
        n129 = Initialize Array(0.0 ("element"), w48) -> (w39:dbl[])
        n130 = call <vilib>:"Send Local Messages.vi"("message queue in"=w36, "message names"=w42, "message values"=w41, "error in"=w45) -> ("error out"=w44:errorcluster)  [unwired: 9 in, 2 out]
        n131 = RT FIFO Write(0:w40, 1:w39, 3:w44) -> (11:w46:errorcluster)  [unwired: 2 in, 3 out]
      }
    }
    n132 = call "Global Stop Actions.vi"("Command"=Stop_Global_Commands."Read", "error in (no error)"=w19, "Stop on Error?"=FALSE, "vi reference"=w18) -> ("error out"=w16:errorcluster, "Latched Stop"=w15:bool)  [unwired: 5 in, 1 out]
    n133 = call "Report Error to Process.vi"("Error"=w16, "This VI"=w17) -> ()  [unwired: 10 in]
  }
  "error out" <- w7
